vi "RichToFlatnixnet_grpc_DbMergeRequest.vi"(5 "OutputClusterType":T1, 11 "InputCluster":T4) -> (3 "OutputCluster":T1)   [LabVIEW 2025, in "xnet-grpc_client.lvlib"]
uses:
  xnet-grpc_client.lvlib
  nixnet_grpc_DbMergeRequest.ctl
  nixnet_grpc_DbMergeRequest_copy_mode_enum/nixnet_grpc_DbMergeRequest_copy_mode_enum.lvclass
  nidevice_grpc_Session.ctl
  nixnet_grpc_DbMergeRequest_Flat.ctl
  nidevice_grpc_Session_Flat.ctl
  nixnet_grpc_CopyMode.ctl
  nixnet_grpc_DbMergeRequest_copy_mode_enum/nixnet_grpc_DbMergeRequest_copy_mode_enum.lvclass/nixnet_grpc_DbMergeRequest_copy_mode_enum.ctl
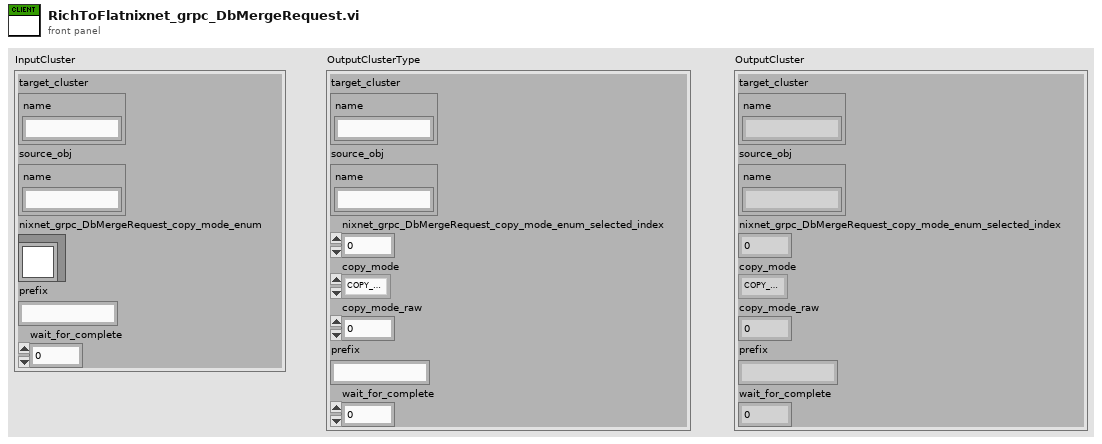
[diagram p1: front panel]
types:
  T1 = typedef "xnet-grpc_client.lvlib/nixnet_grpc_DbMergeRequest_Flat.ctl" = cluster{"target_cluster":T2, "source_obj":T2, "nixnet_grpc_DbMergeRequest_copy_mode_enum_selected_index":i32, "copy_mode":T3, "copy_mode_raw":u32, "prefix":string, "wait_for_complete":u32}
  T2 = typedef "xnet-grpc_client.lvlib/nidevice_grpc_Session_Flat.ctl" = cluster{"name":string}
  T3 = typedef "xnet-grpc_client.lvlib/nixnet_grpc_CopyMode.ctl" = enum32{"COPY_MODE_DB_MERGE_COPY_USE_SOURCE", "COPY_MODE_DB_MERGE_COPY_USE_TARGET", "COPY_MODE_DB_MERGE_MERGE_USE_SOURCE", "COPY_MODE_DB_MERGE_MERGE_USE_TARGET"}
  T4 = typedef "xnet-grpc_client.lvlib/nixnet_grpc_DbMergeRequest.ctl" = cluster{"target_cluster":T5, "source_obj":T5, "nixnet_grpc_DbMergeRequest_copy_mode_enum":refnum<class "nixnet_grpc_DbMergeRequest_copy_mode_enum.lvclass">, "prefix":string, "wait_for_complete":u32}
  T5 = typedef "xnet-grpc_client.lvlib/nidevice_grpc_Session.ctl" = cluster{"name":string}
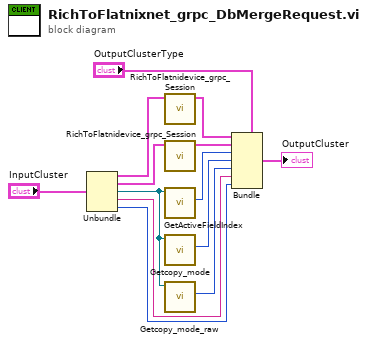
[diagram p0: block diagram]
diagram:
  n1 = Unbundle "Unbundle"("InputCluster") -> ("target_cluster"=w10:T5, "source_obj"=w8:T5, "nixnet_grpc_DbMergeRequest_copy_mode_enum"=w6:refnum<class "nixnet_grpc_DbMergeRequest_copy_mode_enum.lvclass">, "prefix"=w2:string, "wait_for_complete"=w1:u32)
  n2 = call "RichToFlatnidevice_grpc_Session.vi"("InputCluster"=w10) -> ("OutputCluster"=w9:T2)  [unwired: 10 in]
  n3 = call "RichToFlatnidevice_grpc_Session.vi"("InputCluster"=w8) -> ("OutputCluster"=w7:T2)  [unwired: 10 in]
  n4 = call "GetActiveFieldIndex.vi"("OneOfTemplate in"=w6) -> ("Active Field Index"=w5:i32)  [unwired: 8 in, 2 out]
  n5 = call "Getcopy_mode.vi"("OneOfTemplate in"=w6) -> ("Get_Val"=w4:T3)  [unwired: 8 in, 2 out]
  n6 = call "Getcopy_mode_raw.vi"("OneOfTemplate in"=w6) -> ("Get_Val"=w3:u32)  [unwired: 8 in, 2 out]
  n7 = Bundle "Bundle"(cluster="OutputClusterType", "target_cluster"=w9, "source_obj"=w7, "nixnet_grpc_DbMergeRequest_copy_mode_enum_selected_index"=w5, "copy_mode"=w4, "copy_mode_raw"=w3, "prefix"=w2, "wait_for_complete"=w1) -> (→"OutputCluster":T1)
